vi "Configure_power_analyzer.vi"(4 "Negative Voltage Limit (0.0 volts)":dbl format="%^.3e", 6 "Priority (1: Voltage)":i32, 7 "Positive Voltage Limit  (5.0 V)":dbl, 9 "Channel Name (1)":string, 10 "Range (0.0)":dbl, 11 "VISA Refnum in":refnum<visa-resource-name>) -> (0 "error out":errorcluster, 3 "VISA Refnum out":refnum<visa-resource-name>)   [LabVIEW 2015]
uses:
  <instrlib>/Agilent N6700 Series/Agilent N6700 Series.lvlib
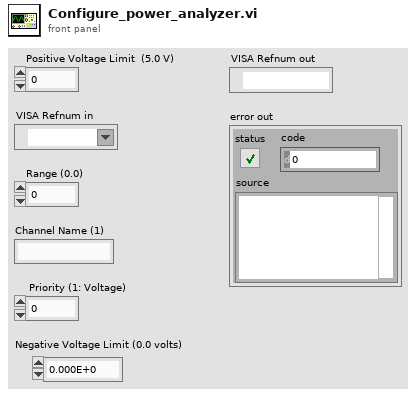
[diagram p1: front panel]
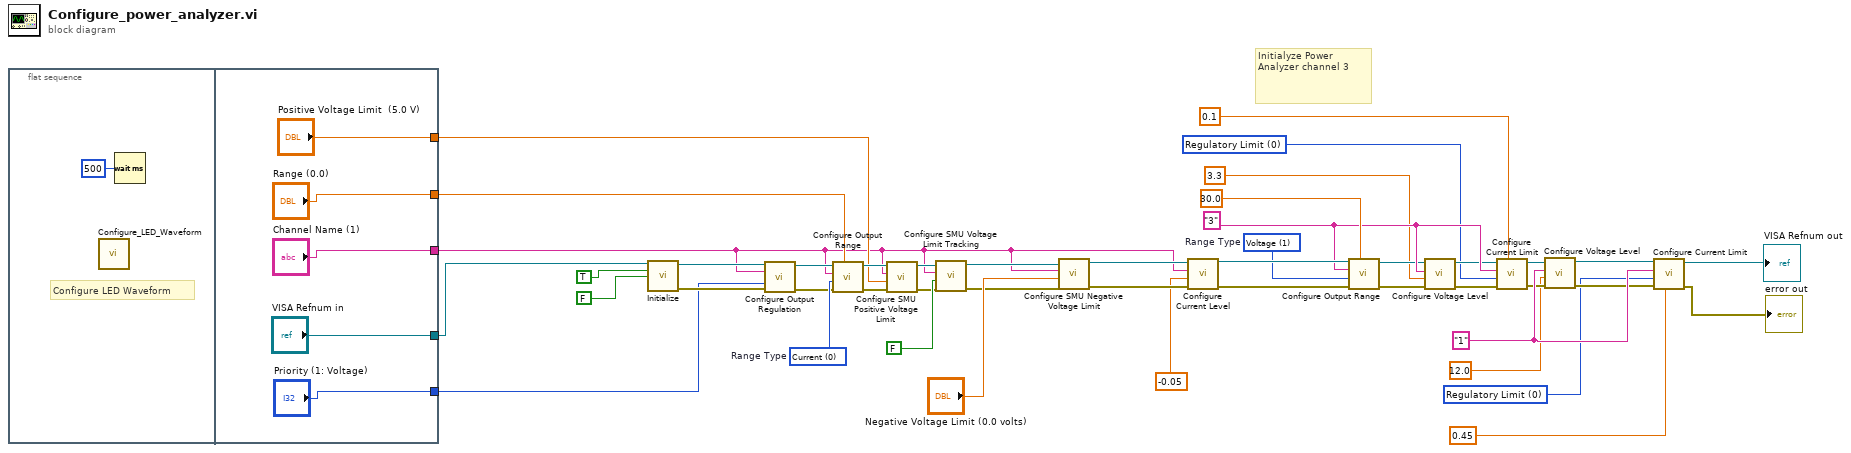
[diagram p0: block diagram]
diagram:
  w43 = "1" ("Channel Name (1)")
  w37 = 0 items=["Regulatory Limit", "Trip Limit"] ("Behavior (0: Regulatory Limit)")
  w34 = "3" ("Channel Name (1)")
  w27 = 0 items=["Regulatory Limit", "Trip Limit"] ("Behavior (0: Regulatory Limit)")
  w31 = 1 items=["Voltage"=1, "Current"=0]  # Range Type
  w16 = 0 items=["Voltage"=1, "Current"=0]  # Range Type
  # "Initialyze Power Analyzer channel 3"
  n1 = flat-sequence {
    tunnel: ["Positive Voltage Limit  (5.0 V)"] -> w8
    tunnel: ["Range (0.0)"] -> w7
    tunnel: ["Channel Name (1)"] -> w6
    tunnel: ["VISA Refnum in"] -> w5
    tunnel: ["Priority (1: Voltage)"] -> w4
    frame #0 {
      # "Configure LED Waveform"
      n2 = call "Configure_LED_Waveform.vi"() -> ()  [unwired: 12 in]
      n3 = Wait (ms)(milliseconds to wait=u32 500) -> ()  [unwired: 1 out]
    }
    frame #1 {
    }
  }
  n4 = call <instrlib>:"Initialize.vi"("VISA resource name"=w5, "ID Query? (T: Yes)"=TRUE ("Reset? (T: Yes)"), "Reset? (T: Yes)"=FALSE) -> ("VISA resource name out"=w24:refnum<visa-resource-name>, "error out"=w25:errorcluster)  [unwired: 11 in]
  n5 = call <instrlib>:"Configure Output Regulation.vi"("VISA resource name"=w24, "Channel Name (1)"=w6, "Output Regulation Priority (1: Voltage)"=w4, "error in (no error)"=w25) -> ("VISA resource name out"=w14:refnum<visa-resource-name>, "error out"=w13:errorcluster)  [unwired: 10 in]
  n6 = call <instrlib>:"Configure Output Range.vi"("Range (0.0)"=w7, "error in (no error)"=w13, "Range Type (1: Voltage)"=w16, "Channel Name (1)"=w6, "VISA resource name"=w14) -> ("error out"=w11:errorcluster, "VISA resource name out"=w12:refnum<visa-resource-name>)  [unwired: 5 in]
  n7 = call <instrlib>:"Configure SMU Positive Voltage Limit.vi"("error in (no error)"=w11, "Positive Voltage Limit (0.0 volts)"=w8, "Channel Name (1)"=w6, "VISA resource name"=w12) -> ("error out"=w9:errorcluster, "VISA resource name out"=w10:refnum<visa-resource-name>)  [unwired: 6 in]
  n8 = call <instrlib>:"Configure SMU Voltage Limit Tracking.vi"("error in (no error)"=w9, "Enable Voltage Limit Tracking (False)"=FALSE, "Channel Name (1)"=w6, "VISA resource name"=w10) -> ("error out"=w20:errorcluster, "VISA resource name out"=w19:refnum<visa-resource-name>)  [unwired: 6 in]
  n9 = call <instrlib>:"Configure SMU Negative Voltage Limit.vi"("error in (no error)"=w20, "Negative Voltage Limit (0.0 volts)"="Negative Voltage Limit (0.0 volts)", "Channel Name (1)"=w6, "VISA resource name"=w19) -> ("error out"=w23:errorcluster, "VISA resource name out"=w22:refnum<visa-resource-name>)  [unwired: 6 in]
  n10 = call <instrlib>:"Configure Current Level.vi"("error in (no error)"=w23, "Level  (0.0 A)"=-0.05, "Channel Name (1)"=w6, "VISA resource name"=w22) -> ("error out"=w45:errorcluster, "VISA resource name out"=w44:refnum<visa-resource-name>)  [unwired: 6 in]
  n11 = call <instrlib>:"Configure Output Range.vi"("Range (0.0)"=30.0, "error in (no error)"=w45, "Range Type (1: Voltage)"=w31, "Channel Name (1)"=w34, "VISA resource name"=w44) -> ("error out"=w29:errorcluster, "VISA resource name out"=w30:refnum<visa-resource-name>)  [unwired: 5 in]
  n12 = call <instrlib>:"Configure Voltage Level.vi"("error in (no error)"=w29, "Level  (0.0 volts)"=3.3, "Channel Name (1)"=w34, "VISA resource name"=w30) -> ("error out"=w33:errorcluster, "VISA resource name out"=w32:refnum<visa-resource-name>)  [unwired: 6 in]
  n13 = call <instrlib>:"Configure Current Limit.vi"("Limit (0.0 amps)"=0.1, "error in (no error)"=w33, "Behavior (0: Regulatory Limit)"=w27, "Channel Name (1)"=w34, "VISA resource name"=w32) -> ("error out"=w41:errorcluster, "VISA resource name out"=w42:refnum<visa-resource-name>)  [unwired: 5 in]
  n14 = call <instrlib>:"Configure Voltage Level.vi"("error in (no error)"=w41, "Level  (0.0 volts)"=12.0, "Channel Name (1)"=w43, "VISA resource name"=w42) -> ("error out"=w40:errorcluster, "VISA resource name out"=w39:refnum<visa-resource-name>)  [unwired: 6 in]
  n15 = call <instrlib>:"Configure Current Limit.vi"("Limit (0.0 amps)"=0.45, "error in (no error)"=w40, "Behavior (0: Regulatory Limit)"=w37, "Channel Name (1)"=w43, "VISA resource name"=w39) -> ("error out"=→"error out":errorcluster, "VISA resource name out"=→"VISA Refnum out":refnum<visa-resource-name>)  [unwired: 5 in]
